vi "MSRV_ParsingInputJSON.vi"(8 "Error In":errorcluster, 11 "data":string) -> (0 "Error Out":errorcluster, 1 "command":string, 2 "name":string, 3 "Mode out":enum16{"get", "set", "close", "Init", "Check"}(ring))   [LabVIEW 2018]
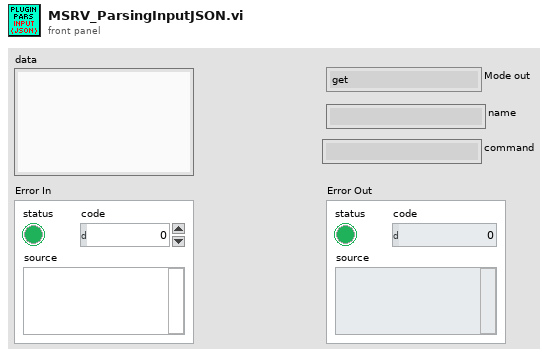
[diagram p1: front panel]
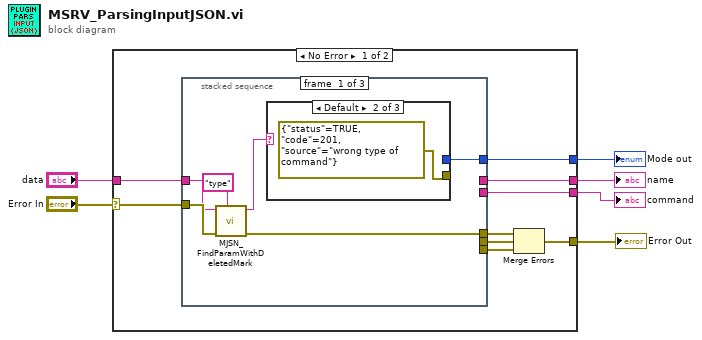
[diagram p0: block diagram]
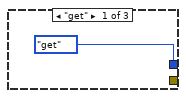
[diagram p2: hidden frame]
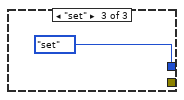
[diagram p3: hidden frame]
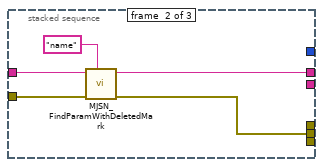
[diagram p4: hidden frame]
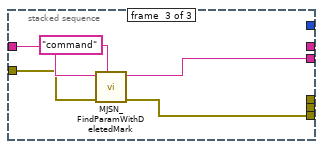
[diagram p5: hidden frame]
diagram:
  n1 = case shown="No Error" "Error In" {
    selector: "Error In" -> [w15 w35]
    tunnel: "data" -> [w13 _]
    tunnel: [w12 _] -> w5
    tunnel: [w7 w35] -> w3
    tunnel: [w14 _] -> w2
    tunnel: [w11 _] -> w1
    frame No Error {
      n2 = stacked-sequence {
        tunnel: w15 -> [w21 w29 w33]
        tunnel: [w20 _ _] -> w14
        tunnel: w13 -> [w18 w27 w34]
        tunnel: [_ _ w32] -> w12
        tunnel: [_ w26 _] -> w11
        tunnel: [w17 _ _] -> w10
        tunnel: [_ w25 _] -> w9
        tunnel: [_ _ w31] -> w8
        frame #0 {
          n3 = call "MJSN_FindParamWithDeletedMark.vi"("Name"="type" ("name"), "Error in (no error)"=w21, "Data"=w18) -> ("Error out"=w17:errorcluster, "Param output"=w16:string)  [unwired: 6 in, 1 out]
          n4 = case shown="Default" w16 {
            tunnel: [enum16{"get", "set", "close", "Init", "Check"}."get" ("Mode") _ enum16{"get", "set", "close", "Init", "Check"}."set" ("Mode")] -> w20
            tunnel: [_ errorcluster {"status"=TRUE, "code"=201, "source"="wrong type of command"} ("Error") _] -> _
            frame "get" {
            }
            frame Default {
            }
            frame "set" {
            }
          }
        }
        frame #1 {
          n5 = call "MJSN_FindParamWithDeletedMark.vi"("Name"="name" ("name"), "Error in (no error)"=w29, "Data"=w27) -> ("Error out"=w25:errorcluster, "Param output"=w26:string)  [unwired: 6 in, 1 out]
        }
        frame #2 {
          n6 = call "MJSN_FindParamWithDeletedMark.vi"("Name"="command" ("name"), "Error in (no error)"=w33, "Data"=w34) -> ("Error out"=w31:errorcluster, "Param output"=w32:string)  [unwired: 6 in, 1 out]
        }
      }
      n7 = Merge Errors(w10, w9, w8) -> (w7:errorcluster)
    }
    frame Error {
    }
  }
  "command" <- w5
  "Mode out" <- w2
  "Error Out" <- w3
  "name" <- w1
